vi "get_all_menu_items.vi"(6 "MenuItem Collection reference":refnum<k24>, 8 "error in (no error)":errorcluster, 9 "MenuItem references in":refnum<k24>[](array[refnum]), 11 "BalloonNotifier in":refnum<class "BalloonNotifier.lvclass">) -> (0 "error out":errorcluster, 3 "BalloonNotifier out":refnum<class "BalloonNotifier.lvclass">, 4 "MenuItem references out":refnum<k24>[](array[refnum]))   [LabVIEW 2010, in "BalloonNotifier.lvclass"]
uses:
  BalloonNotifier.lvclass
  System.Windows.Forms
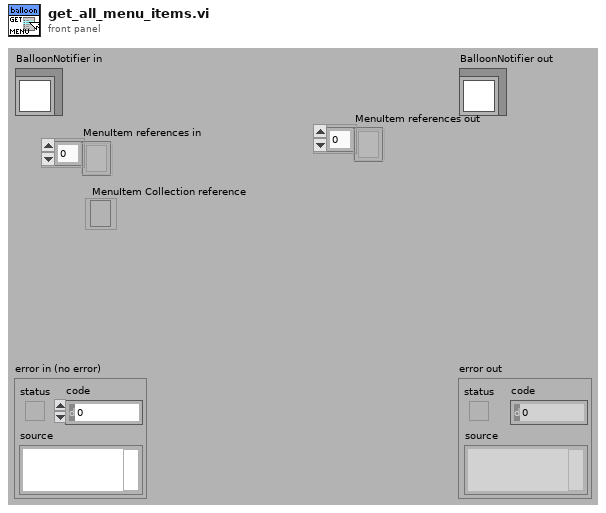
[diagram p1: front panel]
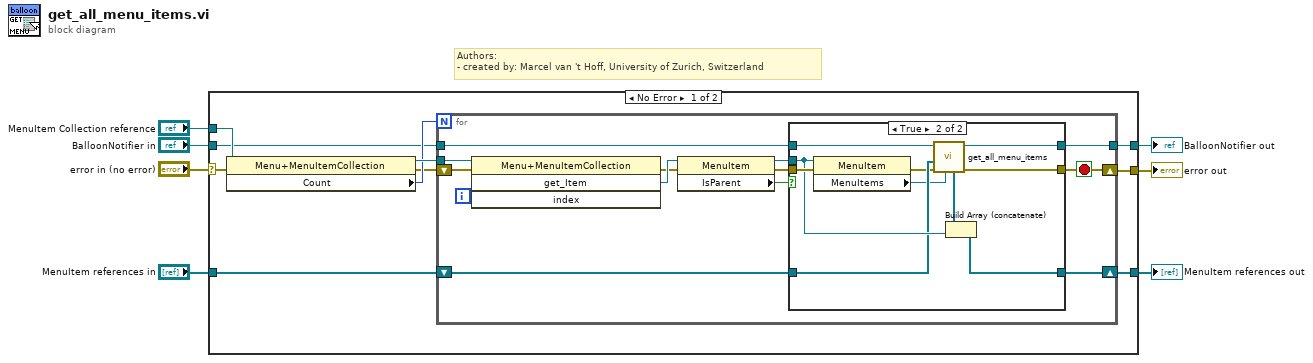
[diagram p0: block diagram]
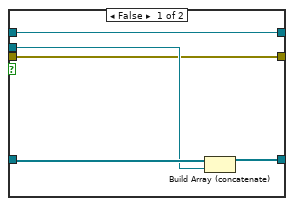
[diagram p2: hidden frame]
diagram:
  # "Authors: \n- created by: Marcel van 't Hoff, University of Zurich, Switzerland"
  n1 = case shown="No Error" "error in (no error)" {
    selector: "error in (no error)" -> [w10 w48]
    tunnel: "MenuItem references in" -> [w15 w47]
    tunnel: "MenuItem Collection reference" -> [w14 _]
    tunnel: [w13 w47] -> w1
    tunnel: [w11 w48] -> w4
    tunnel: [w8 w46] -> w3
    tunnel: "BalloonNotifier in" -> [w9 w46]
    frame No Error {
      n2 = property class="Menu+MenuItemCollection"(reference=w14, error in=w10) -> (reference out=w17:refnum<k24>, error out=w12:errorcluster, "Count"=w16:i32)
      n3 = for {
        N: w16 -> [_]
        tunnel: w17 -> [w30]
        shift-right: [w27] -> w13
        shift-left: w15 -> [w26]
        shift-right: [w21] -> w11
        shift-left: w12 -> [w24]
        tunnel: w9 -> [w19]
        tunnel: [w18] -> w8
        i -> [w20]
        stop <- w21 stop-if-true
        n4 = invoke class="Menu+MenuItemCollection" method="get_Item"(reference=w30, error in=w24, "index"=w20) -> (error out=w23:errorcluster, "get_Item"=w28:refnum<k24>)  [unwired: 1 in, 2 out]
        n5 = property class="MenuItem"(reference=w28, error in=w23) -> (reference out=w25:refnum<k24>, error out=w22:errorcluster, "IsParent"=w29:bool)
        n6 = case shown="True" w29 {
          tunnel: [w35 w43] -> w27
          tunnel: w26 -> [w34 w42]
          tunnel: w25 -> [w33 w44]
          tunnel: w22 -> [w32 w45]
          tunnel: [w32 w39] -> w21
          tunnel: w19 -> [w31 w37]
          tunnel: [w31 w36] -> w18
          frame False {
            n7 = Build Array (concatenate)(w34, w33) -> (w35:refnum<k24>[])
          }
          frame True {
            n8 = property class="MenuItem"(reference=w44, error in=w45) -> (error out=w38:errorcluster, "MenuItems"=w40:refnum<k24>)  [unwired: 1 out]
            n9 = call-dynamic "get_all_menu_items.vi"("MenuItem Collection reference"=w40, "error in (no error)"=w38, "MenuItem references in"=w42, "BalloonNotifier in"=w37) -> ("error out"=w39:errorcluster, "BalloonNotifier out"=w36:refnum<class "BalloonNotifier.lvclass">, "MenuItem references out"=w41:refnum<k24>[])  [unwired: 5 in]
            n10 = Build Array (concatenate)(w41, w44) -> (w43:refnum<k24>[])
          }
        }
      }
    }
    frame Error {
    }
  }
  "error out" <- w4
  "BalloonNotifier out" <- w3
  "MenuItem references out" <- w1
